vi "HomographyCtoXY.vi"(2 "Y":dbl, 3 "X":dbl, 4 "C":T1) -> (0 "Y":dbl, 1 "X":dbl)   [LabVIEW 2015]
uses:
  <vilib>/Analysis/Matrix/Datatypes/RealMatrix.ctl
  <vilib>/Analysis/baseanly.llb/Real A x B.vi
  <vilib>/Analysis/Matrix/Numeric/Conversions/Matrix To Array - RM.vi
  <vilib>/Analysis/NI_AALBase.lvlib
  <vilib>/Analysis/Matrix/NI_Matrix.lvlib
panel:
  out "A x B":T1
  out "appended array":T1
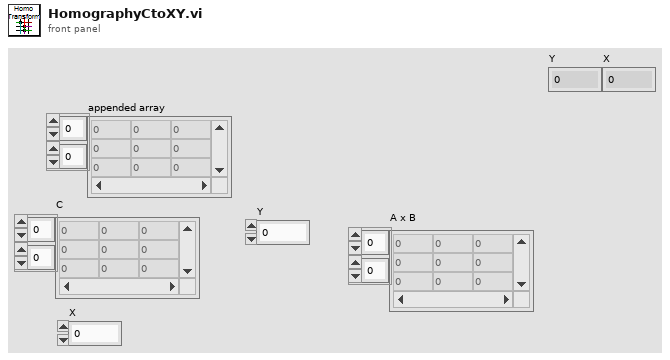
[diagram p1: front panel]
types:
  T1 = typedef "NI_Matrix.lvlib/RealMatrix.ctl" = dbl[][]
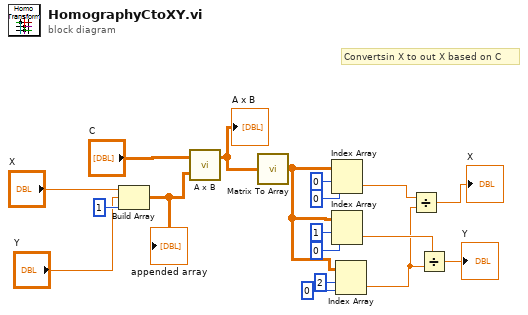
[diagram p0: block diagram]
diagram:
  # "Convertsin X to out X based on C"
  n1 = Build Array("X", "Y", 1 ("index (row)")) -> (w17:T1)
  "appended array" <- w17
  n2 = call-poly <vilib>:"A x B.vi"("B"=w17, "A"="C") -> ("A x B"=w16:T1)  [unwired: 1 out]
  "A x B" <- w16
  n3 = call-poly <vilib>:"Matrix To Array.vi"("Real Matrix"=w16) -> ("Real 2D Array"=w12:dbl[][])
  n4 = Index Array(array=w12, index (row)=0, index (col)=0 ("disabled index (col)")) -> (element=w8:dbl)
  n5 = Index Array(array=w12, index (row)=1, index (col)=0 ("disabled index (col)")) -> (element=w7:dbl)
  n6 = Index Array(array=w12, index (row)=2, index (col)=0 ("disabled index (col)")) -> (element=w6:dbl)
  n7 = Divide(x=w8, y=w6) -> (x/y=→"X":dbl)
  n8 = Divide(x=w7, y=w6) -> (x/y=→"Y":dbl)
